vi "Get Status Pointer.vi"(8 "error in (no error)":errorcluster, 11 "Framework Status in":refnum<class "Framework Status.lvclass">) -> (0 "error out":errorcluster, 2 "status pointer":refnum<class "Status Pointer.lvclass">, 3 "Framework Status out":refnum<class "Framework Status.lvclass">)   [LabVIEW 2017, in "DSF Core.lvlib" / "Framework Status.lvclass"]
uses:
  Framework Status.lvclass
  Status/Status Pointer.lvclass
  Framework Status.lvclass/Framework Status.ctl
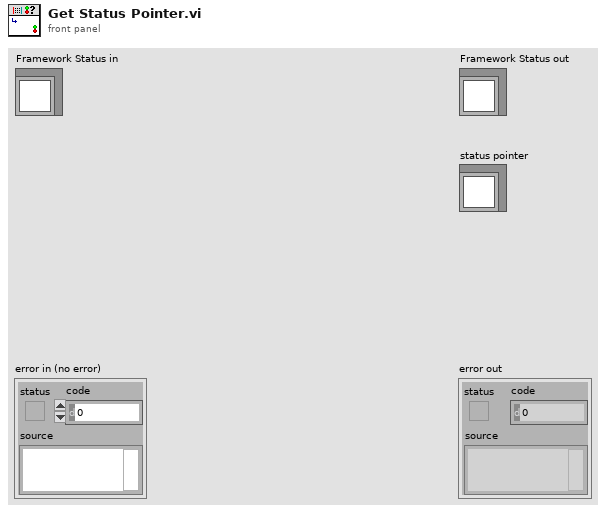
[diagram p1: front panel]
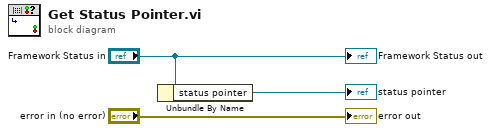
[diagram p0: block diagram]
diagram:
  n1 = Unbundle By Name("Framework Status in") -> ("status pointer"=→"status pointer":refnum<class "Status Pointer.lvclass">)
  "error out" <- "error in (no error)"
  "Framework Status out" <- "Framework Status in"
